vi "Refresh Tree.vi"(8 "error in":errorcluster, 9 "VIs (including clones)":string[](array[string]), 11 "ConfigInfo in":T1={"Data Tree Ref"=refnum, "FP Ref"=refnum, "Column Data Type"=[], "AppInst"=refnum, "Search Clones Up To"=100, "SortOptions"={"Col.pri"=0, "RevDir.pri"=FALSE, "Col.sec"=0, "RevDir.sec"=FALSE}, "Group/Flat (0:group)"=FALSE, "CollapsedNodes"=[], "Show/Hide Cols"=[], "Filtered Paths"=[], "Folder View"=FALSE, "File Extension Filters"=[], "Filter Global VIs"=FALSE, "Tracked Item Tags"=[]}) -> (0 "error out":errorcluster, 3 "ConfigInfo out":T1={"Data Tree Ref"=refnum, "FP Ref"=refnum, "Column Data Type"=[], "AppInst"=refnum, "Search Clones Up To"=100, "SortOptions"={"Col.pri"=0, "RevDir.pri"=FALSE, "Col.sec"=0, "RevDir.sec"=FALSE}, "Group/Flat (0:group)"=FALSE, "CollapsedNodes"=[], "Show/Hide Cols"=[], "Filtered Paths"=[], "Folder View"=FALSE, "File Extension Filters"=[], "Filter Global VIs"=FALSE, "Tracked Item Tags"=[]})   [LabVIEW 2013]
uses:
  Controls_LVTM/LVTM_Config_Info.ctl
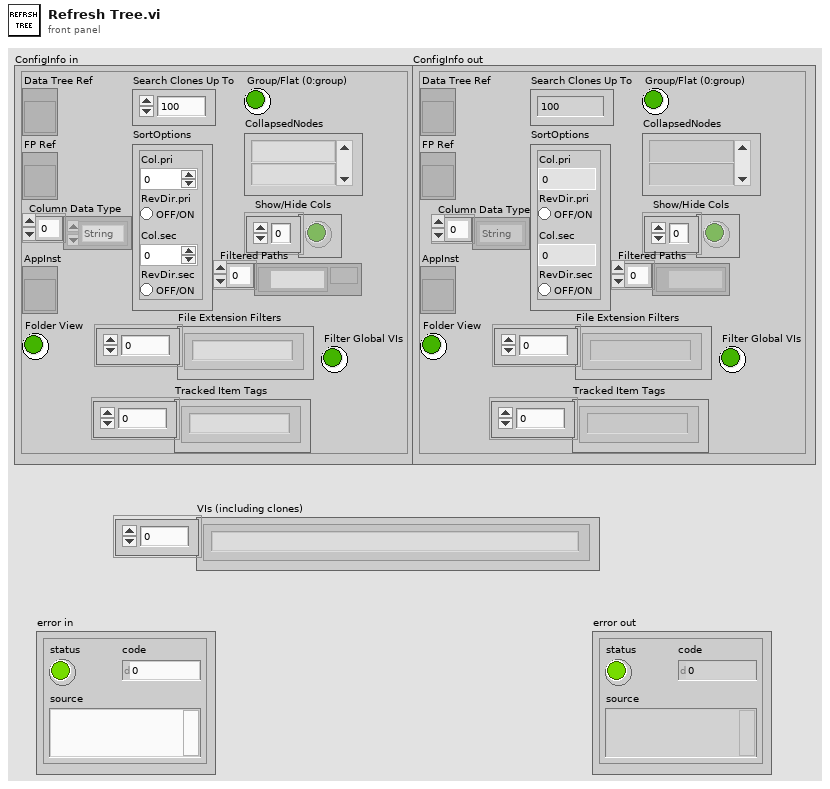
[diagram p1: front panel]
types:
  T1 = typedef "LVTM_Config_Info.ctl" = cluster{"Data Tree Ref":refnum<vi>, "FP Ref":refnum<vi>, "Column Data Type":enum16{"String", "Numeric"}[], "AppInst":refnum<vi>, "Search Clones Up To":i32, "SortOptions":cluster{"Col.pri":i32, "RevDir.pri":bool, "Col.sec":i32, "RevDir.sec":bool}, "Group/Flat (0:group)":bool, "CollapsedNodes":string[], "Show/Hide Cols":bool[], "Filtered Paths":path[], "Folder View":bool, "File Extension Filters":string[], "Filter Global VIs":bool, "Tracked Item Tags":string[]}
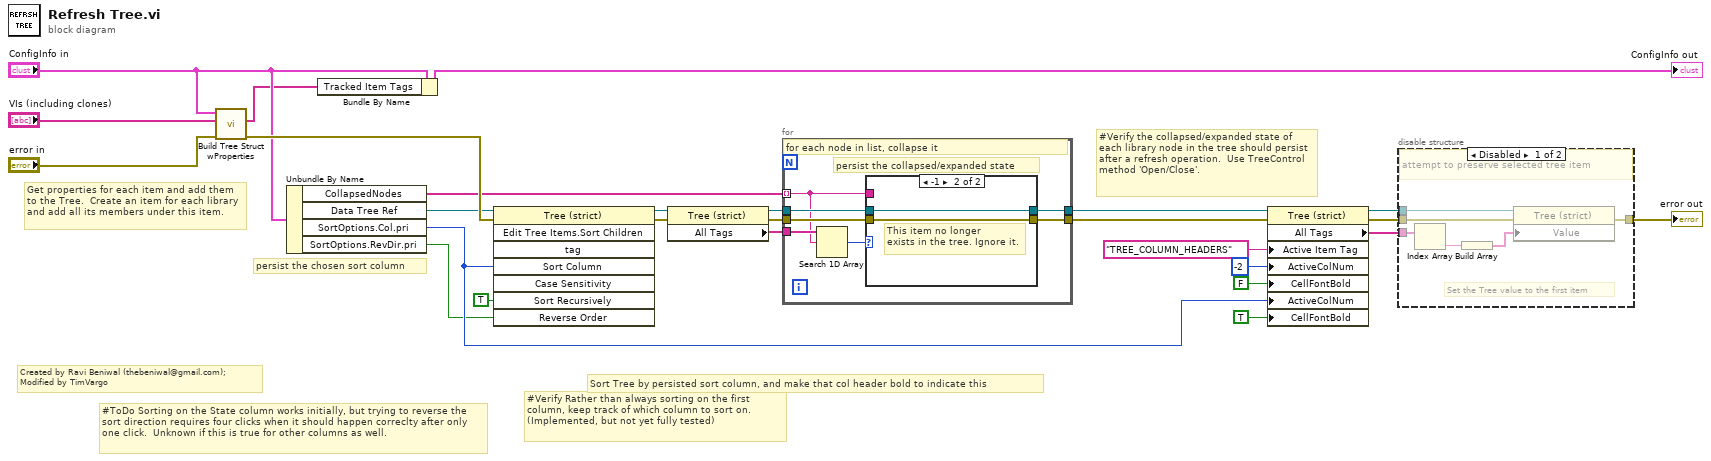
[diagram p0: block diagram]
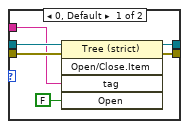
[diagram p2: hidden frame]
diagram:
  # "#ToDo Sorting on the State column works initially, but trying to reverse the sort direction requires four clicks when it should happen correclty after only one click.  Unknown if this is true for other columns as well."
  # "Get properties for each item and add them to the Tree.  Create an item for each library and add all its members under this item."
  # "#Verify the collapsed/expanded state of each library node in the tree should persist after a refresh operation.  Use TreeControl method 'Open/Close'."
  # "persist the chosen sort column"
  # "Created by Ravi Beniwal (thebeniwal@gmail.com);\nModified by TimVargo"
  # "#Verify Rather than always sorting on the first column, keep track of which column to sort on.\n(Implemented, but not yet fully tested)"
  # "Sort Tree by persisted sort column, and make that col header bold to indicate this"
  n1 = call "Build Tree Struct wProperties.vi"("error in"="error in", "VIs (including clones)"="VIs (including clones)", "ConfigInfo in"="ConfigInfo in") -> ("error out"=w16:errorcluster, "Item Tags"=w6:string[])  [unwired: 7 in]
  n2 = Unbundle By Name("ConfigInfo in") -> ("CollapsedNodes"=w8:string[], "Data Tree Ref"=w14:refnum<vi>, "SortOptions.Col.pri"=w12:i32, "SortOptions.RevDir.pri"=w11:bool)
  n3 = Bundle By Name(cluster="ConfigInfo in", "Tracked Item Tags"=w6) -> (→"ConfigInfo out":T1)
  n4 = invoke on="Invoke Node" class="Tree (strict)" method="Edit Tree Items.Sort Children"(reference=w14, error in=w16, "Sort Column"=w12, "Sort Recursively"=TRUE ("Sort Recursively?"), "Reverse Order"=w11) -> (reference out=w5:refnum<vi>, error out=w3:errorcluster)  [unwired: 3 in, 6 out]
  n5 = property class="Tree (strict)"(reference=w5, error in=w3) -> (reference out=w4:refnum<vi>, error out=w2:errorcluster, "All Tags"=w1:string[])
  n6 = for {
    tunnel: w4 -> [w33]
    tunnel: [w32] -> w10
    tunnel: [w31] -> w9
    tunnel: w2 -> [w30]
    tunnel: w8 -> [w28] mode=indexing
    tunnel: w1 -> [w29]
    # "persist the collapsed/expanded state"
    # "for each node in list, collapse it"
    n7 = Search 1D Array(1D array=w29, element=w28) -> (index of element=w27:i32)  [unwired: 1 in]
    n8 = case shown="-1" w27 {
      tunnel: w33 -> [w39 w41]
      tunnel: [w38 w41] -> w32
      tunnel: [w37 w40] -> w31
      tunnel: w30 -> [w36 w40]
      tunnel: w28 -> [w34 _]
      frame 0, Default {
        n9 = invoke on="Invoke Node" class="Tree (strict)" method="Open/Close.Item"(reference=w39, error in=w36, "tag"=w34, "Open"=FALSE ("Open?")) -> (reference out=w38:refnum<vi>, error out=w37:errorcluster)  [unwired: 1 in, 3 out]
      }
      frame -1 {
        # "This item no longer\nexists in the tree. Ignore it."
      }
    }
  }
  n10 = property class="Tree (strict)"(reference=w10, error in=w9, "Active Item Tag"="TREE_COLUMN_HEADERS" ("Active Item:Tag"), "ActiveColNum"=-2 ("Active Cell:Active Column Number"), "CellFontBold"=FALSE ("Active Cell:Cell Font:Bold"), "ActiveColNum"=w12, "CellFontBold"=TRUE ("Active Cell:Cell Font:Bold")) -> (reference out=w19:refnum<vi>, error out=w18:errorcluster, "All Tags"=w17:string[])
  n11 = disable-structure shown="Disabled" {
    disable-tunnel: w19 -> [w46 _]
    disable-tunnel: w18 -> [w45 w48]
    disable-tunnel: w17 -> [w44 _]
    disable-tunnel: [w42 w48] -> w15
    frame Disabled {
      # "Set the Tree value to the first item"
      # "attempt to preserve selected tree item"
      n12 = Index Array(array=w44) -> (element=w47:string)  [unwired: 1 in]
      n13 = Build Array(w47) -> (w43:string[])
      n14 = property class="Tree (strict)"(reference=w46, error in=w45, "Value"=w43) -> (error out=w42:errorcluster)  [unwired: 1 out]
    }
    frame Enabled {
    }
  }
  "error out" <- w15
